vi "Data Classification.vi"   [LabVIEW 2020]
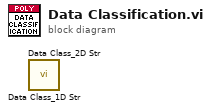
[diagram p0: block diagram]
diagram:
  n1 = call "Data Class_1D Str.vi"() -> ()  [unwired: 10 in, 2 out]
  n2 = call "Data Class_2D Str.vi"() -> ()  [unwired: 7 in, 5 out]
